vi "X-_Commands.vi"(4 "Channel Name":string, 5 "R/W":enum16{"READ", "WRITE"}(ring), 6 "Port Name":string, 7 "String Value":string, 8 "Numeric Value":dbl format="%.2f", 9 "COMMAND":T1, 10 "Address":u8) -> (0 "String Reply":string, 2 "Numeric Reply":dbl format="%.2f")   [LabVIEW 2010]
uses:
  X-_commands.ctl
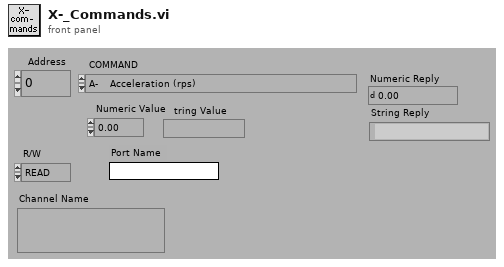
[diagram p1: front panel]
types:
  T1 = typedef "X-_commands.ctl" = enum16{"A-    Acceleration (rps)", "B-    Buffer Status", "C-    Continue", "CG-  Correction Gain", "CR-  Cariage Return", "D-    Distance (pulses)", "DB-  Dead Band (encoder steps)", "DW- Deadband Window (encoder steps)", "E-    Enable Communications", "ER-  Encoder Resolution (steps/rev)", "F-    Disable Communications", "FS-  Encoder Functions Report", "FSA- Incremental/Absolute (0/1)", "FSB- Motor/Encoder Step Mode (0/1)", "FSC- Enable/Disable Position Maint. (1/0)", "FSD- Stop/Continue on Stall (1/0)", "FSE- Activate o/p1 on Stall (1/0)", "FSF- Stop Motion on Trig3 (1/0)", "FSG- Activate o/p2 in Deadband (1/0)", "FSH- Enable Stall Detect (1/0)", "G- Go", "GH- Go Home and Zero (+/-V)", "^H- Delete ", "H- Direction Reverse/CCW/CW (0,1,2)", "IS- Input Status", "K- Kill", "L- Loop (n)", "LD- Limit DISABLE (0-none,1-CW,2-CCW,3-Both)", "LF- Line Feed", "MC- Mode Continuous", "MN- Mode Normal", "MPA- Motor Postion Absolute", "MPI- Motor Position Incremental", "MR- Motor Resolution (Drive Steps/rev)", "N- End of Loop", "O- Output (00,01,10,11)", "OS- Report Homing Setup", "OSA- NO/NC Limits (1/0)", "OSB- Back Up to Home/Edge? (0/1)", "OSC- NO/NC Home Switch (1/0)", "OSD- Enable Encoder Z for Home (0/1)", "OSH- Reference Edge for Home CW/CCW (0/1)", "PR- Report ABSOLUTE Position", "PS- Pause until Continue", "PX- Report Absolute ENCODER Position", "PZ- Zero Absolute Counter", "\"- Quote (17 ASCII +Space)", "Q- Enter/Exit Velocity Profiling (1/0)", "R- Request Indexer Status", "RA- Report Limit Switch Status", "RB- Report Loop, Pause, Shutdown, Trigger Status", "RC- Report Closed Loop Status", "RM- Velocity Streaming Rate Multiplier (000-FFF)", "RV- Report Revision Level", "S- Controlled Stop", "SN- Debounce (1-1000ms)", "SS- Report Software Switch Status", "SSA- Disable RS232 Echo (1/0)", "SSG- Clear/Save Command Buffer on Limit (0/1)", "SSH- Clear/Save Command Buffer on Stop (0/1)", "ST- Shutdown (1/0)", "SV- Servoing Setting (0,1,2,3)", "T- Time Delay (0.01-99999.99)", "TR- Wait for Trigger High/Low/Ignore (1/0/X)", "TS- Report Trigger Status", "U- Pause after Move Until Continue", "V- Velocity (0.01-50.00 revs/sec)", "W1- Report Relative Position <Signed Binary>", "W3- Report Relative Position <Hexadecimal>", "Y- Abort Loop at N", "Z-    Reset to Defaults", "#-    Disable/Set Soft Addresses (0/1-255)"}
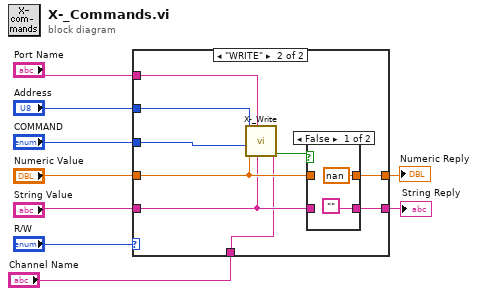
[diagram p0: block diagram]
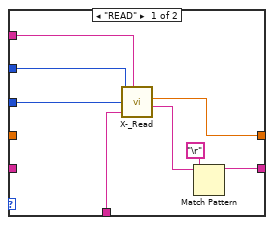
[diagram p2: hidden frame]
diagram:
  n1 = case shown="\"WRITE\"" "R/W" {
    tunnel: "Port Name" -> [w10 w26]
    tunnel: "COMMAND" -> [w17 w24]
    tunnel: "Address" -> [w16 w25]
    tunnel: [w15 w23] -> w6
    tunnel: [w13 w21] -> w5
    tunnel: "Numeric Value" -> [_ w22]
    tunnel: "String Value" -> [_ w20]
    tunnel: "Channel Name" -> [w11 w19]
    frame "READ" {
      n2 = call "X-_Read.vi"("Address"=w16, "Port Name"=w10, "COMMAND"=w17, "Channel Name"=w11) -> ("Numeric Reply"=w15:dbl, "String Reply"=w14:string)  [unwired: 4 in, 1 out]
      n3 = Match Pattern(string=w14, regular expression="\r") -> (before substring=w13:string)  [unwired: 1 in, 3 out]
    }
    frame "WRITE" {
      n4 = call "X-_Write.vi"("Channel Name"=w19, "String to write"=w20, "Port Name"=w26, "Value"=w22, "COMMAND"=w24, "Address"=w25) -> ("Good Echo"=w18:bool)  [unwired: 5 in]
      n5 = case shown="False" w18 {
        tunnel: [nan ("Numeric Value") w30] -> w23
        tunnel: w22 -> [_ w30]
        tunnel: ["" w29] -> w21
        tunnel: w20 -> [_ w29]
        frame False {
        }
        frame True {
        }
      }
    }
  }
  "String Reply" <- w5
  "Numeric Reply" <- w6
